vi "Ex-01 Acq Single point.vi"() -> ()   [LabVIEW 2012]
doc: "© Copyright M. Ferrari 2012 \nSgl. Point Analog Acq. Template"
uses:
  <vilib>/DAQmx/read.llb/DAQmx Read (Analog DBL 1Chan 1Samp).vi
  <vilib>/DAQmx/create/channels.llb/DAQmx Create Channel (AI-Voltage-Basic).vi
panel:
  in  "Mul Factor":dbl(knob)=1.0 scale=0.0..100.0
  in  "Delay":u32=100
  out "Wfrm Chart":dbl(graph)=1.0589674728404055
  in  "min":dbl=-5.0 format="%0.2f"
  in  "max":dbl=5.0 format="%0.2f"
  in  "stop":bool
  in  "in conf":i32(ring)=10083 items=["default"=-1, "RSE"=10083, "NRSE"=10078, "Differential"=10106, "Pseudodifferential"=12529]
  in  "physical ch":tag="Dev1/ai0"
  # "RANGE"
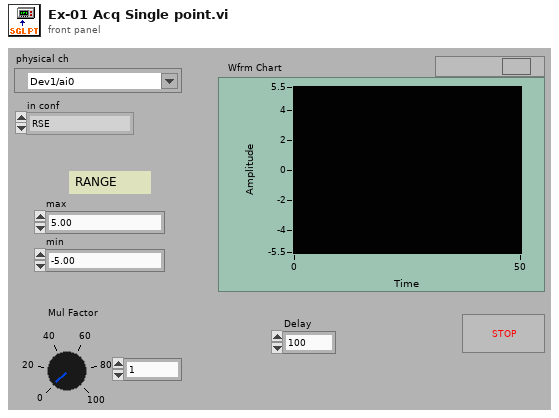
[diagram p1: front panel]
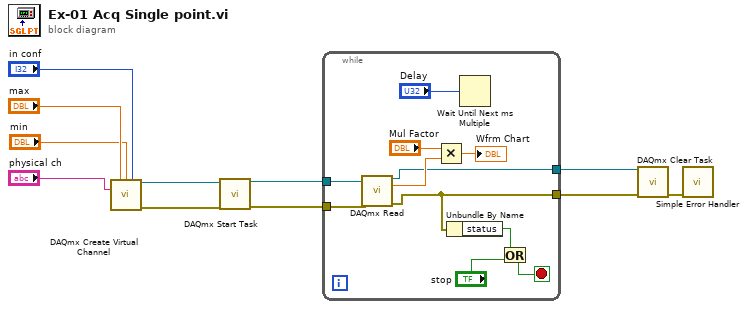
[diagram p0: block diagram]
diagram:
  n1 = call-poly <vilib>:"DAQmx Create Virtual Channel.vi"("maximum value"="max", "minimum value"="min", "input terminal configuration"="in conf", "physical channels"="physical ch") -> ("task out"=w6:refnum<k21>, "error out"=w5:errorcluster)  [unwired: 5 in, 5 out]
  n2 = call <vilib>:"DAQmx Start Task.vi"("task/channels in"=w6, "error in"=w5) -> ("task out"=w2:refnum<k21>, "error out"=w1:errorcluster)  [unwired: 12 out]
  n3 = while {
    tunnel: [w14] -> w4
    tunnel: [w17] -> w3
    tunnel: w2 -> [w16]
    tunnel: w1 -> [w15]
    stop <- w19 stop-if-true
    n4 = call-poly <vilib>:"DAQmx Read.vi"("task/channels in"=w16, "error in"=w15) -> ("task out"=w17:refnum<k21>, "data"=w18:dbl, "error out"=w14:errorcluster)  [unwired: 11 out]
    n5 = Multiply(x="Mul Factor", y=w18) -> (x*y=→"Wfrm Chart":dbl)
    n6 = Unbundle By Name(w14) -> ("status"=w13:bool)
    n7 = Wait Until Next ms Multiple(millisecond multiple="Delay") -> ()  [unwired: 1 out]
    n8 = Or(x=w13, y="stop") -> (x .or. y?=w19:bool)
  }
  n9 = call <vilib>:"DAQmx Clear Task.vi"("task in"=w3, "error in"=w4) -> ("error out"=w11:errorcluster)  [unwired: 13 out]
  n10 = call <vilib>:"Simple Error Handler.vi"("error in (no error)"=w11) -> ()  [unwired: 1 in, 8 out]
